vi "SRQ Mask (GPIB).vi"(7 "Read Value? (F)":bool, 8 "error in (no error)":errorcluster, 10 "SRQ Mask (Scan Finished)":T1={"Parameter Changed from Front Panel"=FALSE, "Data Ready"=FALSE, "Scan Finished"=TRUE, "Counter Overrun"=FALSE, "Rate Error"=FALSE, "Recall Error"=FALSE, "Service Request"=FALSE, "Command Error"=FALSE}, 11 "VISA resource name":refnum<visa-resource-name>) -> (0 "error out":errorcluster, 2 "SRQ Mask":T1, 3 "VISA resource name out":refnum<visa-resource-name>)   [LabVIEW 2013, in "SRS SR400.lvlib"]
doc: "<B>SV { m }</B>\n\nIf m is included, the SV command sets the GPIB SRQ (service request) mask to the value m (0-255). If m is absent, the value of the SRQ mask is returned. The SV command may only be sent via the GPIB interface."
uses:
  <instrlib>/SRS SR400/SRS SR400.lvlib
  <instrlib>/SRS SR400/Public/Typedefs/Status Byte.ctl
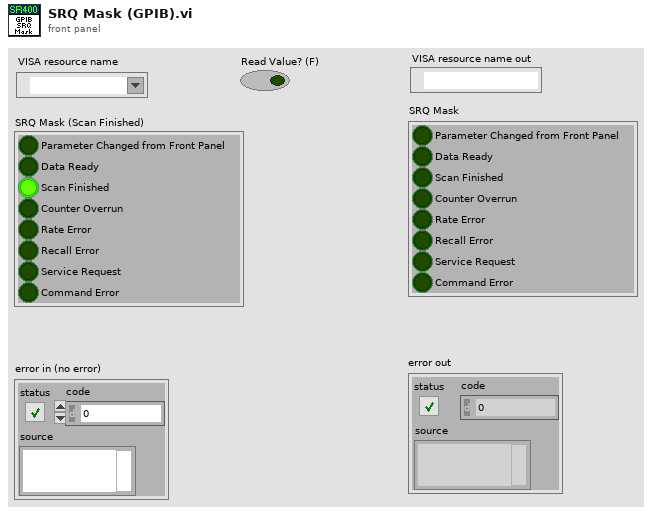
[diagram p1: front panel]
types:
  T1 = typedef "SRS SR400.lvlib/Status Byte.ctl" = cluster{"Parameter Changed from Front Panel":bool, "Data Ready":bool, "Scan Finished":bool, "Counter Overrun":bool, "Rate Error":bool, "Recall Error":bool, "Service Request":bool, "Command Error":bool}
  T2 = cluster{"Boolean array[0]":bool, "Boolean array[1]":bool, "Boolean array[2]":bool, "Boolean array[3]":bool, "Boolean array[4]":bool, "Boolean array[5]":bool, "Boolean array[6]":bool, "Boolean array[7]":bool}
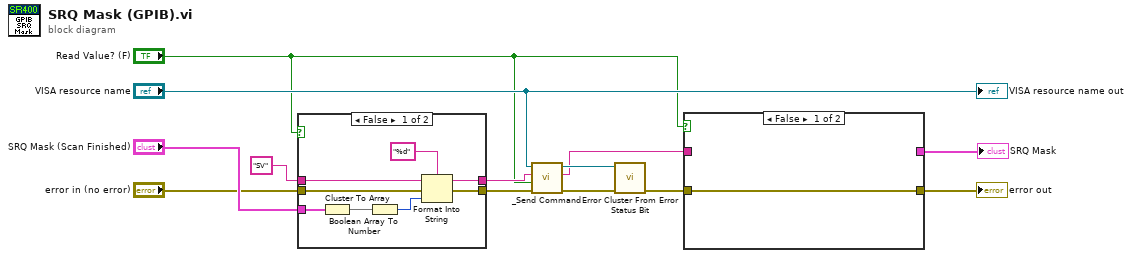
[diagram p0: block diagram]
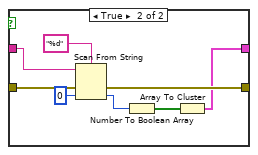
[diagram p2: hidden frame]
diagram:
  n1 = case shown="False" "Read Value? (F)" {
    tunnel: "SRQ Mask (Scan Finished)" -> [w21 _]
    tunnel: "SV" ("initial string") -> [w19 w22]
    tunnel: [w17 w22] -> w11
    tunnel: "error in (no error)" -> [w15 w23]
    tunnel: [w14 w23] -> w6
    frame False {
      n2 = Cluster To Array(cluster=w21) -> (array=w16:bool[])
      n3 = Boolean Array To Number(Boolean array=w16) -> (number=w18:u8)
      n4 = Format Into String(format string="%d", initial string=w19, error in=w15, w18) -> (resulting string=w17:string, error out=w14:errorcluster)
    }
    frame True {
    }
  }
  n5 = call <instrlib>:"_Send Command.vi"("error in (no error)"=w6, "Read Value? (F)"="Read Value? (F)", "Command"=w11, "VISA resource name"="VISA resource name") -> ("error out"=w8:errorcluster, "Response"=w2:string, "VISA resource name out"=w9:refnum<visa-resource-name>)  [unwired: 5 out]
  n6 = call <instrlib>:"Error Cluster From Error Status Bit.vi"("error in (no error)"=w8, "VISA resource name"=w9) -> ("error out"=w5:errorcluster)  [unwired: 8 in, 1 out]
  n7 = case shown="False" "Read Value? (F)" {
    tunnel: w5 -> [w24 w32]
    tunnel: [w24 w31] -> w3
    tunnel: w2 -> [_ w30]
    tunnel: [_ w25] -> w1
    frame False {
    }
    frame True {
      n8 = Scan From String(format string="%d", input string=w30, error in=w32, default 1=u8 0 ("default value 1")) -> (error out=w31:errorcluster, output 1=w27:u8)  [unwired: 1 in, 2 out]
      n9 = Number To Boolean Array(number=w27) -> (Boolean array=w26:bool[])
      n10 = Array To Cluster(array=w26) -> (cluster=w25:T2)
    }
  }
  "error out" <- w3
  "SRQ Mask" <- w1
  "VISA resource name out" <- "VISA resource name"
